vi "MotionProfileBuffer.vi"(8 "error in (no error)":errorcluster, 11 "CTRE Drive in":refnum<class "CTRE Drive.lvclass">) -> (0 "error out":errorcluster, 3 "CTRE Drive out":refnum<class "CTRE Drive.lvclass">)   [LabVIEW 2019, in "Drive.lvlib" / "CTRE Drive.lvclass"]
uses:
  CTRE Drive.lvclass
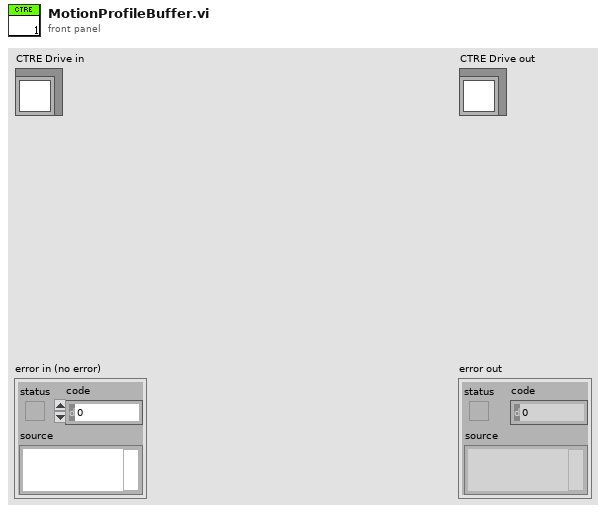
[diagram p1: front panel]
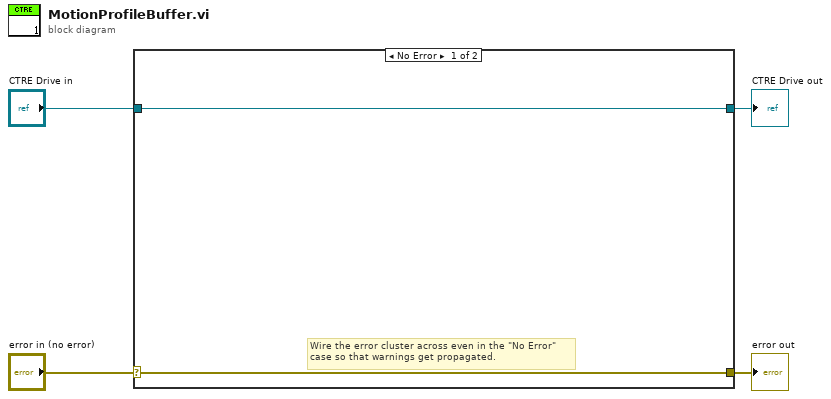
[diagram p0: block diagram]
diagram:
  n1 = case shown="No Error" "error in (no error)" {
    selector: "error in (no error)" -> [w5 w8]
    tunnel: [w5 w8] -> w3
    tunnel: [w6 w7] -> w1
    tunnel: "CTRE Drive in" -> [w6 w7]
    frame No Error {
      # "Wire the error cluster across even in the \"No Error\"\ncase so that warnings get propagated."
    }
    frame Error {
    }
  }
  "error out" <- w3
  "CTRE Drive out" <- w1
